vi "TCP_R.vi"(8 "error in":errorcluster, 9 "timeout ms":i32, 11 "connection ID":refnum<k5>) -> (0 "error out":errorcluster, 2 "data out":string, 3 "connection ID out":refnum<k5>)   [LabVIEW 2012]
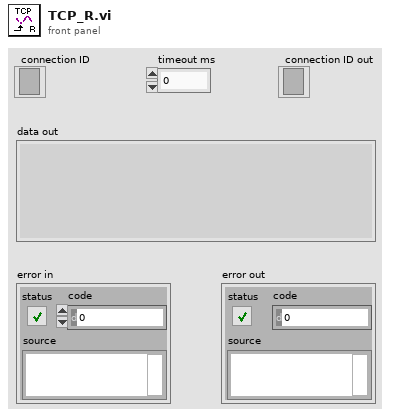
[diagram p1: front panel]
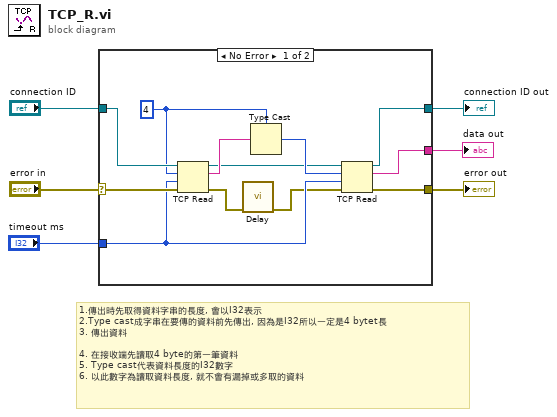
[diagram p0: block diagram]
diagram:
  # "1.傳出時先取得資料字串的長度, 會以I32表示\n2.Type cast成字串在要傳的資料前先傳出, 因為是I32所以一定是4 bytet長\n3. 傳出資料\n\n4. 在接收端先讀取4 byte的第一筆資料\n5. Type cast代表資料長度的I32數字\n6. 以此數字為讀取資料長度, 就不會有漏掉或多取的資料"
  n1 = case shown="No Error" "error in" {
    selector: "error in" -> [w18 w20]
    tunnel: [w8 w20] -> w4
    tunnel: "connection ID" -> [w17 w19]
    tunnel: [w12 w19] -> w3
    tunnel: "timeout ms" -> [w11 _]
    tunnel: [w7 _] -> w1
    frame No Error {
      w15 = 4 ("bytes to read")
      n2 = TCP Read(connection ID=w17, bytes to read=w15, error in (no error)=w18, 9:w11) -> (connection ID out=w13:refnum<k5>, data out=w16:string, error out=w10:errorcluster)  [unwired: 1 in]
      n3 = call "Delay.vi"("error in"=w10) -> ("error out"=w9:errorcluster)  [unwired: 10 in]
      n4 = Type Cast(type=w15, x=w16) -> (*(type *) &x=w14:i32)
      n5 = TCP Read(connection ID=w13, bytes to read=w14, error in (no error)=w9, 9:w11) -> (connection ID out=w12:refnum<k5>, data out=w7:string, error out=w8:errorcluster)  [unwired: 1 in]
    }
    frame Error {
    }
  }
  "error out" <- w4
  "connection ID out" <- w3
  "data out" <- w1
